vi "Get_VI_Path.vi"(2 "error in":errorcluster, 3 "VI name (no .vi)":string) -> (0 "error out":errorcluster, 1 "File Path":path)   [LabVIEW 2021]
uses:
  Project_References_Global.vi
  <vilib>/Utility/error.llb/Error Cluster From Error Code.vi
  <vilib>/ErrorRing/Error Ring.xnode
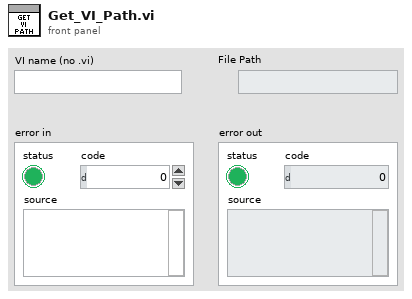
[diagram p1: front panel]
types:
  T1 = cluster{"VI Name":string, "String Path":string}[]
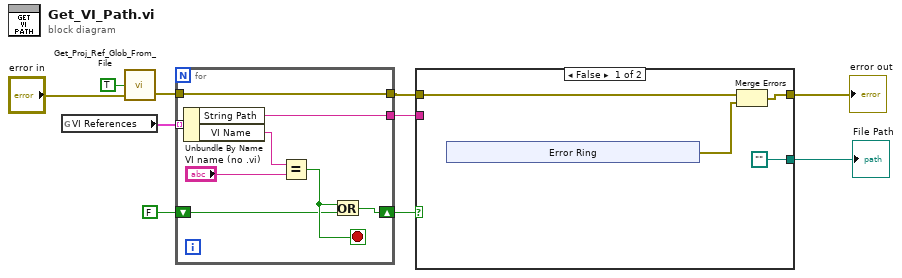
[diagram p0: block diagram]
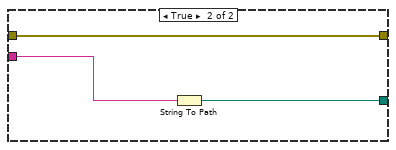
[diagram p2: hidden frame]
diagram:
  n1 = global read "Project_References_Global.vi" "VI References"() -> (w9:T1)
  n2 = call "Get_Proj_Ref_Glob_From_File.vi"("error in"="error in", "Get default(?)"=TRUE) -> ("error out"=w7:errorcluster)  [unwired: 1 in, 1 out]
  n3 = for {
    tunnel: w9 -> [w18] mode=indexing
    shift-right: [w15] -> w6
    shift-left: FALSE -> [w13]
    tunnel: [w12] -> w2
    tunnel: w7 -> [w11]
    tunnel: [w11] -> w3
    stop <- w14 stop-if-true
    n4 = Unbundle By Name(w18) -> ("String Path"=w12:string, "VI Name"=w17:string)
    n5 = Equal?(x=w17, y="VI name (no .vi)") -> (x = y?=w14:bool)
    n6 = Or(x=w14, y=w13) -> (x .or. y?=w15:bool)
  }
  n7 = case shown="False" w6 {
    tunnel: [w22 w30] -> w4
    tunnel: w3 -> [w20 w30]
    tunnel: w2 -> [_ w29]
    tunnel: [path "" w28] -> w1
    frame False {
      n8 = xnode "Error Ring"() -> ("error out"=w21:errorcluster)
      n9 = Merge Errors(w20, w21) -> (w22:errorcluster)
    }
    frame True {
      n10 = String To Path(string=w29) -> (path=w28:path)
    }
  }
  "error out" <- w4
  "File Path" <- w1
